vi "ThermoV_ControlSweep_NoMean_experimentalCODE_dc.vi"() -> ()   [LabVIEW 2013]
panel:
  in  "Operate HVpp\nOutput Timer":bool caption="Reset"
  out "modular 13":dbl
  in  "Number of seconds for \neach HVpp case state":dbl=30.0
  out "Elapsed Time (s)":dbl
  out "DC Value":dbl[](array[numeric]) format="%#.6f"
  in  "Saving Avg?":bool
  in  "Filename":path=path "trial_1.lvm"
  in  "STOP":bool
  in  "Save Waveform":bool
  out "Peak2Peak V":dbl[](array[numeric])
  out "Waveform Chart":dynamicdata(graph)
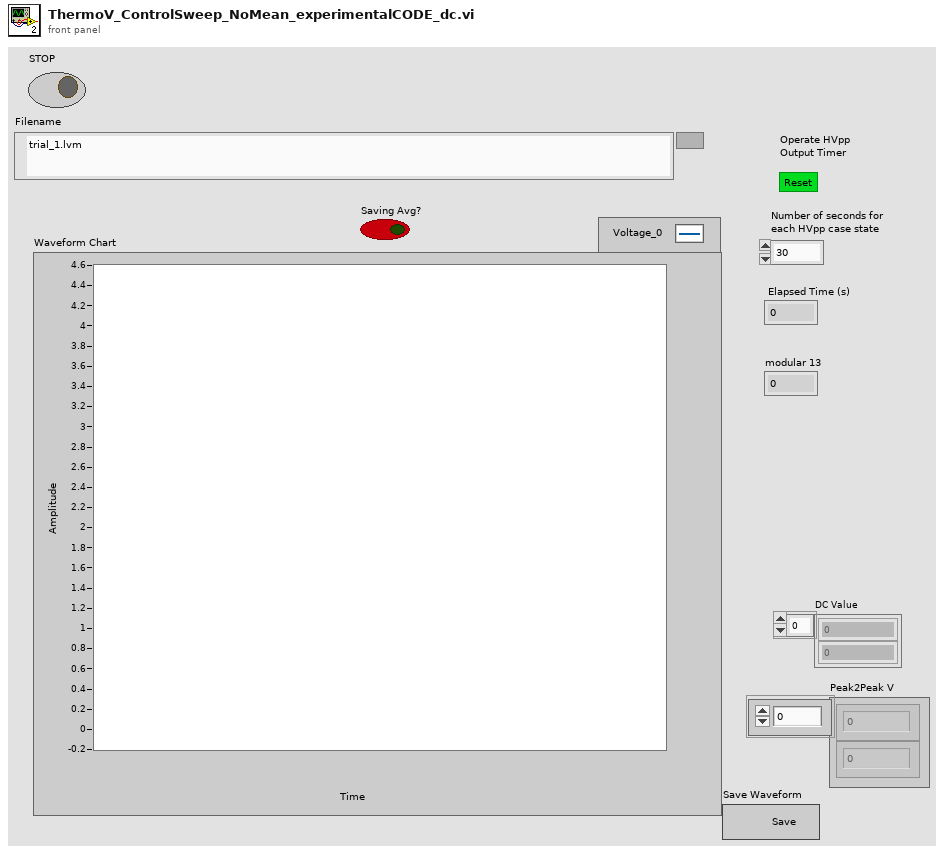
[diagram p1: front panel]
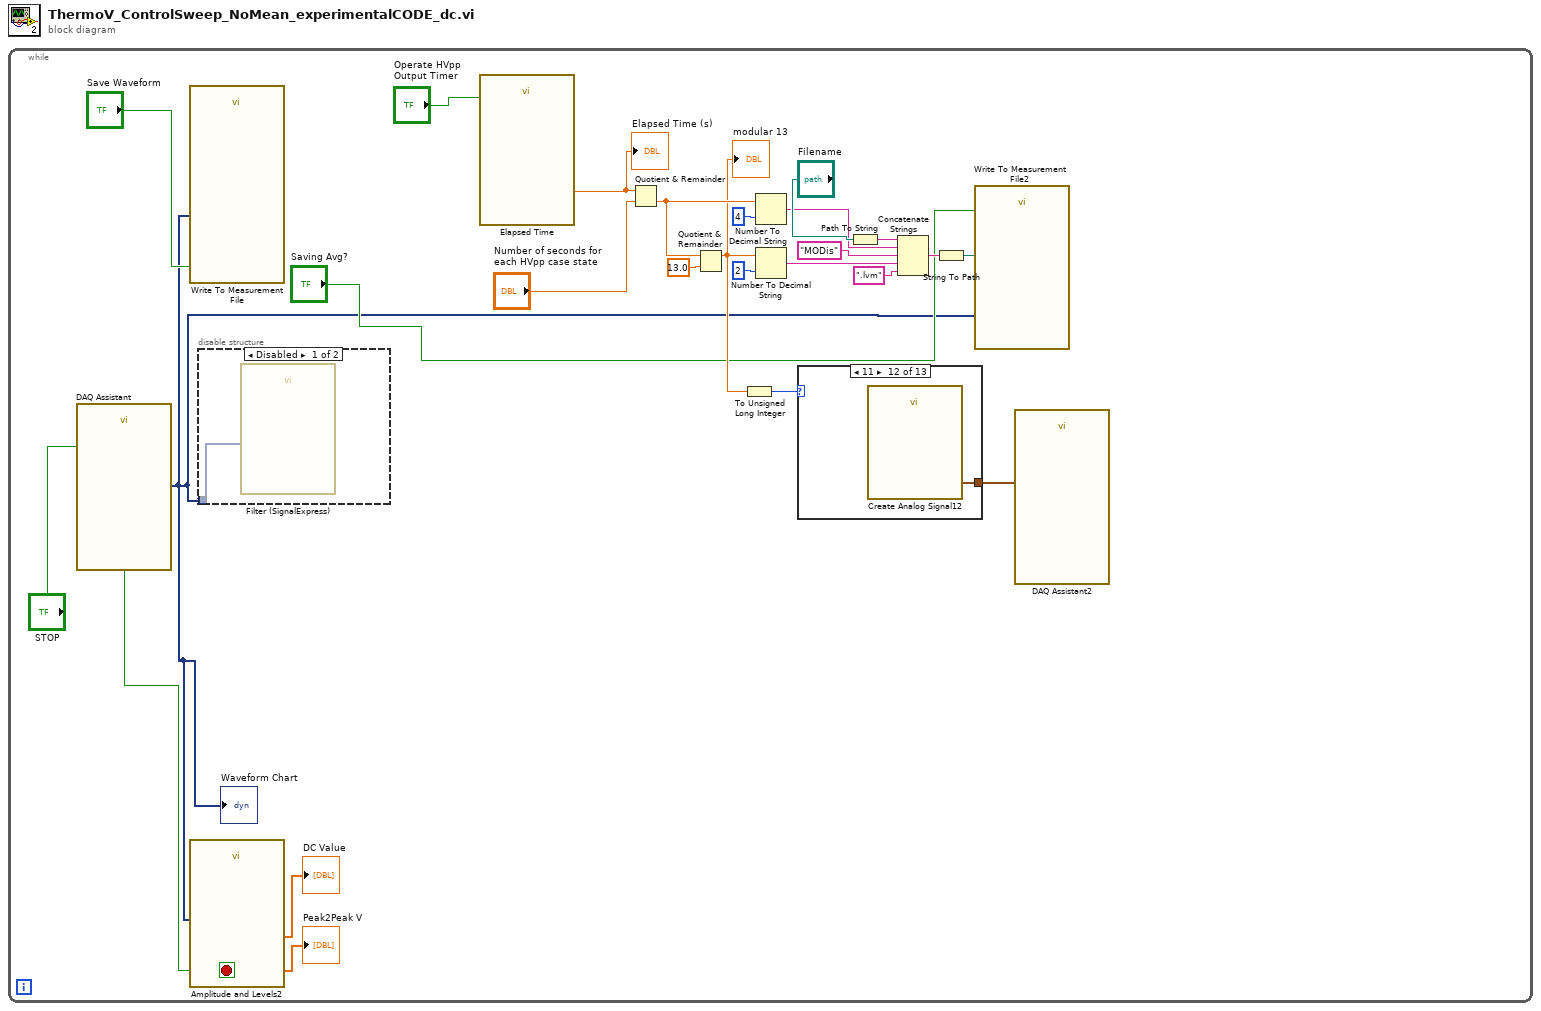
[diagram p0: block diagram]
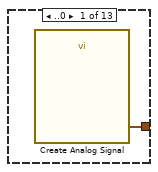
[diagram p3: hidden frame]
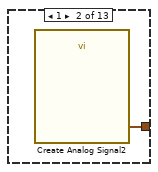
[diagram p4: hidden frame]
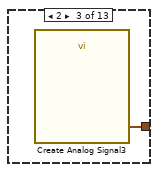
[diagram p5: hidden frame]
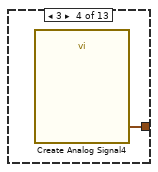
[diagram p6: hidden frame]
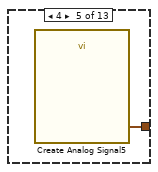
[diagram p7: hidden frame]
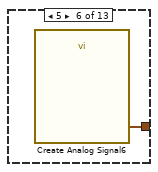
[diagram p8: hidden frame]
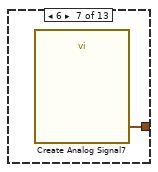
[diagram p9: hidden frame]
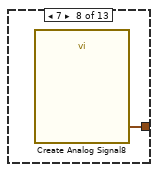
[diagram p10: hidden frame]
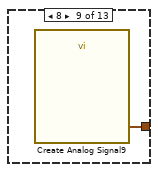
[diagram p11: hidden frame]
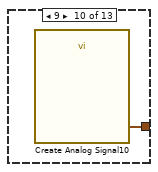
[diagram p12: hidden frame]
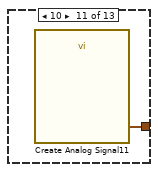
[diagram p13: hidden frame]
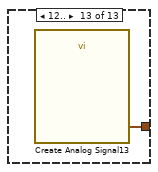
[diagram p14: hidden frame]
diagram:
  n1 = while {
    stop <- w25 stop-if-true
    n2 = call "DAQ Assistant"("stop (F)"="STOP") -> ("data"=w1:dynamicdata, "stopped"=w25:bool)  [unwired: 15 in, 2 out]
    "Waveform Chart" <- w1
    n3 = call "Write To Measurement File"("Signals"=w1, "Enable"="Save Waveform") -> ()  [unwired: 15 in, 3 out]
    n4 = call "Amplitude and Levels2"("input signals"=w1) -> ("dc"=→"DC Value":dbl[], "peak-peak"=→"Peak2Peak V":dbl[])  [unwired: 15 in, 2 out]
    n5 = disable-structure shown="Disabled" {
      disable-tunnel: w1 -> [w26 _]
      frame Disabled {
        n6 = call "Filter (SignalExpress)"("input signal"=w26) -> ()  [unwired: 17 in, 2 out]
      }
      frame Enabled {
      }
    }
    n7 = call "Elapsed Time"("Reset"="Operate HVpp\nOutput Timer") -> ("Elapsed Time (s)"=w18:dbl)  [unwired: 11 in, 7 out]
    "Elapsed Time (s)" <- w18
    n8 = Quotient & Remainder(x=w18, y="Number of seconds for \neach HVpp case state") -> (floor(x/y)=w10:dbl)  [unwired: 1 out]
    n9 = Quotient & Remainder(x=w10, y=13.0) -> (x-y*floor(x/y)=w5:dbl)  [unwired: 1 out]
    "modular 13" <- w5
    n10 = To Unsigned Long Integer(number=w5) -> (unsigned 32bit integer=w19:u32)
    n11 = Number To Decimal String(number=w10, width (-)=i16 4) -> (decimal integer string=w9:string)
    n12 = Number To Decimal String(number=w5, width (-)=i16 2) -> (decimal integer string=w4:string)
    n13 = case shown="11" w19 {
      tunnel: [w27 w28 w29 w30 w31 w32 w33 w34 w35 w36 w37 w38 w39] -> w20
      frame ..0 {
        n14 = call "Create Analog Signal"() -> ("sine wave"=w27:waveform(dbl))  [unwired: 18 in, 1 out]
      }
      frame 1 {
        n15 = call "Create Analog Signal2"() -> ("DC signal"=w28:waveform(dbl))  [unwired: 18 in, 1 out]
      }
      frame 2 {
        n16 = call "Create Analog Signal3"() -> ("sine wave"=w29:waveform(dbl))  [unwired: 18 in, 1 out]
      }
      frame 3 {
        n17 = call "Create Analog Signal4"() -> ("DC signal"=w30:waveform(dbl))  [unwired: 18 in, 1 out]
      }
      frame 4 {
        n18 = call "Create Analog Signal5"() -> ("sine wave"=w31:waveform(dbl))  [unwired: 18 in, 1 out]
      }
      frame 5 {
        n19 = call "Create Analog Signal6"() -> ("DC signal"=w32:waveform(dbl))  [unwired: 18 in, 1 out]
      }
      frame 6 {
        n20 = call "Create Analog Signal7"() -> ("sine wave"=w33:waveform(dbl))  [unwired: 18 in, 1 out]
      }
      frame 7 {
        n21 = call "Create Analog Signal8"() -> ("DC signal"=w34:waveform(dbl))  [unwired: 18 in, 1 out]
      }
      frame 8 {
        n22 = call "Create Analog Signal9"() -> ("sine wave"=w35:waveform(dbl))  [unwired: 18 in, 1 out]
      }
      frame 9 {
        n23 = call "Create Analog Signal10"() -> ("DC signal"=w36:waveform(dbl))  [unwired: 18 in, 1 out]
      }
      frame 10 {
        n24 = call "Create Analog Signal11"() -> ("sine wave"=w37:waveform(dbl))  [unwired: 18 in, 1 out]
      }
      frame 11 {
        n25 = call "Create Analog Signal12"() -> ("DC signal"=w38:waveform(dbl))  [unwired: 18 in, 1 out]
      }
      frame 12.. {
        n26 = call "Create Analog Signal13"() -> ("sine wave"=w39:waveform(dbl))  [unwired: 18 in, 1 out]
      }
    }
    n27 = Path To String(path="Filename") -> (string=w12:string)
    n28 = Concatenate Strings(w12, w9, "MODis" ("string"), w4, ".lvm" ("string")) -> (w14:string)
    n29 = String To Path(string=w14) -> (path=w15:path)
    n30 = call "Write To Measurement File2"("Signals"=w1, "Enable"="Saving Avg?", "Filename"=w15) -> ()  [unwired: 14 in, 3 out]
    n31 = call "DAQ Assistant2"("data"=w20) -> ()  [unwired: 16 in, 3 out]
  }
